vi "Get Writes.vi"(8 "error in":errorcluster, 9 "Value":dbl, 10 "Channel":string, 11 "BufferWritesDBL in":refnum<class "BufferWritesDBL.lvclass">) -> (0 "error out":errorcluster, 2 "Write Buffer":void[](array[numeric]), 3 "BufferWritesDBL out":refnum<class "BufferWritesDBL.lvclass">)   [LabVIEW 2023, in "BufferWritesDBL.lvclass"]
uses:
  BufferWritesDBL.lvclass
  BufferWritesDBL.lvclass/BufferWritesDBL.ctl
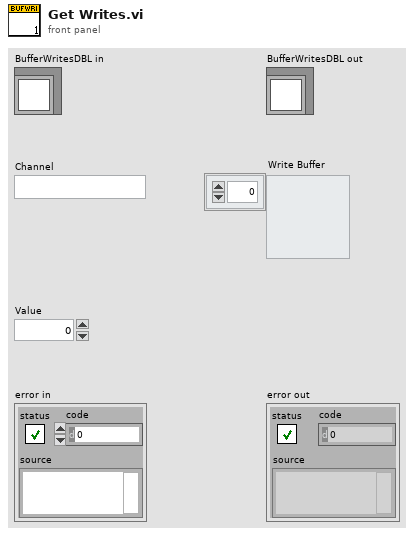
[diagram p1: front panel]
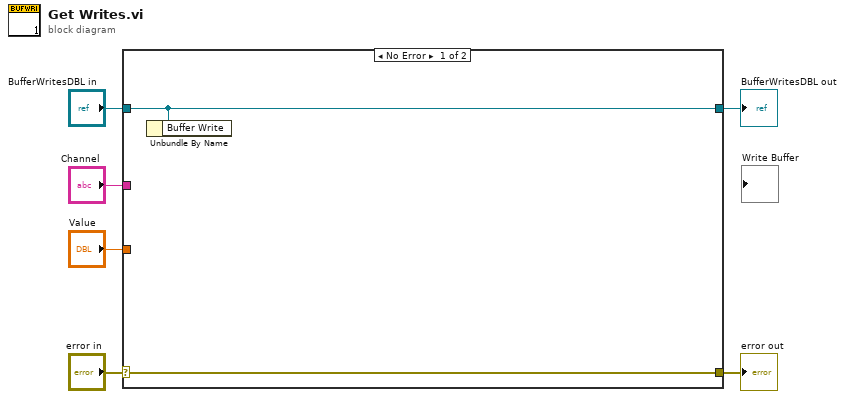
[diagram p0: block diagram]
diagram:
  n1 = case shown="No Error" "error in" {
    selector: "error in" -> [w8 w10]
    tunnel: [w8 w10] -> w5
    tunnel: [w7 w9] -> w3
    tunnel: "BufferWritesDBL in" -> [w7 w9]
    tunnel: "Channel" -> [_ _]
    tunnel: "Value" -> [_ _]
    frame No Error {
      n2 = Unbundle By Name(w7) -> ()  [unwired: 1 out]
    }
    frame Error {
    }
  }
  "error out" <- w5
  "BufferWritesDBL out" <- w3
